vi "dvp Vi Get Hardware Version.vi"(9 "nLength":u32, 10 "HardwareVersion":string, 11 "handle":u32) -> (2 "HardwareVersion out":string, 3 "function return":u32(ring))   [LabVIEW 2018, in "LabViewDVPCamera.lvlib"]
doc: "LabviewDvp2Api dvpStatus dvpViGetHardwareVersion(dvpHandle handle, char *HardwareVersion, dvpUint32 nLength);"
uses:
  LabViewDVPCamera.lvlib
  LabViewDVPCamera/LabViewDVPCamera.dll
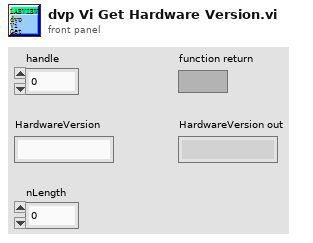
[diagram p1: front panel]
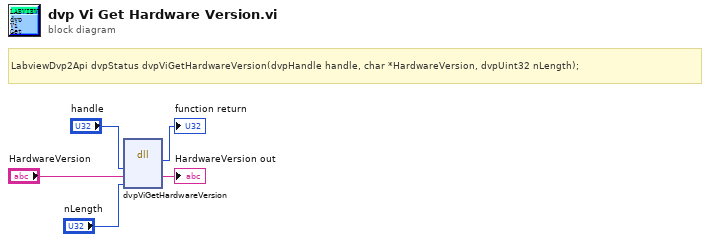
[diagram p0: block diagram]
diagram:
  # "LabviewDvp2Api dvpStatus dvpViGetHardwareVersion(dvpHandle handle, char *HardwareVersion, dvpUint32 nLength);"
  n1 = dll-call lib="C:/Program Files (x86)/DVP2 Labview cn 64/Sample/LabViewDVPCamera/LabViewDVPCamera.*" fn="dvpViGetHardwareVersion"("handle"="handle", "HardwareVersion"="HardwareVersion", "nLength"="nLength") -> (→"function return":u32, "HardwareVersion"=→"HardwareVersion out":string)  [unwired: 5 in, 2 out]
